vi "Configure9211.vi"(7 "Channel Number":i32, 8 "error in (no error)":errorcluster, 10 "Properties":T1[](array[typedef]), 11 "Refnum in":refnum<k21>) -> (0 "error out":errorcluster, 3 "Refnum out":refnum<k21>)   [LabVIEW 2017, in "ScanEngine.lvlib"]
uses:
  <vilib>/addons/InsightCM/Devices/Shared/Common/ScanEngine/ScanEngine.lvlib
  <vilib>/addons/InsightCM/MessageBus/Base/controls/KeyValuePair.ctl
  <resource>/objmgr/cRIO.rc
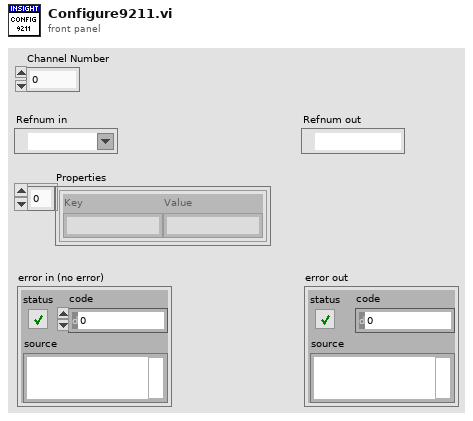
[diagram p1: front panel]
types:
  T1 = typedef "KeyValuePair.ctl" = cluster{"Key":string, "Value":string}
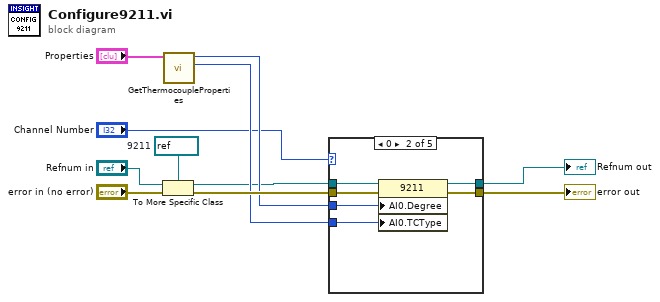
[diagram p0: block diagram]
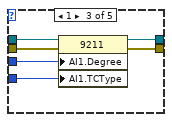
[diagram p3: hidden frame]
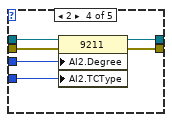
[diagram p4: hidden frame]
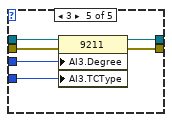
[diagram p5: hidden frame]
diagram:
  w4 = refnum<k21> refnum  # 9211
  n1 = To More Specific Class(target class=w4, reference="Refnum in", error in="error in (no error)") -> (specific class reference=w6:refnum<k21>, error out=w11:errorcluster)
  n2 = call <vilib>:"GetThermocoupleProperties.vi"("Properties"="Properties") -> ("AI Thermocouple type"=w10:u32, "AI degree range"=w9:u32)  [unwired: 9 in]
  n3 = case shown="0" "Channel Number" {
    tunnel: w11 -> [w13 w17 w23 w29 w35]
    tunnel: [w13 w19 w25 w31 w37] -> w1
    tunnel: w6 -> [w12 w18 w24 w30 w36]
    tunnel: w9 -> [_ w16 w22 w28 w34]
    tunnel: w10 -> [_ w15 w21 w27 w33]
    tunnel: [w12 w14 w20 w26 w32] -> w7
    frame -1, Default {
    }
    frame 0 {
      n4 = property class="9211"(reference=w18, error in=w17, "AI0.Degree"=w16, "AI0.TCType"=w15) -> (reference out=w14:refnum<k21>, error out=w19:errorcluster)
    }
    frame 1 {
      n5 = property class="9211"(reference=w24, error in=w23, "AI1.Degree"=w22, "AI1.TCType"=w21) -> (reference out=w20:refnum<k21>, error out=w25:errorcluster)
    }
    frame 2 {
      n6 = property class="9211"(reference=w30, error in=w29, "AI2.Degree"=w28, "AI2.TCType"=w27) -> (reference out=w26:refnum<k21>, error out=w31:errorcluster)
    }
    frame 3 {
      n7 = property class="9211"(reference=w36, error in=w35, "AI3.Degree"=w34, "AI3.TCType"=w33) -> (reference out=w32:refnum<k21>, error out=w37:errorcluster)
    }
  }
  "Refnum out" <- w7
  "error out" <- w1
